vi "SDCP SMF Rx Logger - Test.vi"() -> ()   [LabVIEW 2020]
uses:
  Typedefs/SDCP SMF logger - SMF with timestamp.ctl
  SDCP SMF Rx Logger - FGV - Commands.vi
  Typedefs/SDCP - Serial Port Control - Commands.ctl
panel:
  out "Number of samples for instantaeneous samples":i32
  out "Instantaeneous logged data":T1[](array[typedef])
  out "Elapse time (ms)":u32
  out "Logging started":bool
  out "Number of samples":i32
  in  "Stop logging":bool
  in  "Log interval (ms)":u32
  in  "Number of iterations":i32
  out "Rx data":T1[](array[typedef])
  in  "Baud rate":u32=9600
  in  "COM Port":refnum<visa-resource-name>
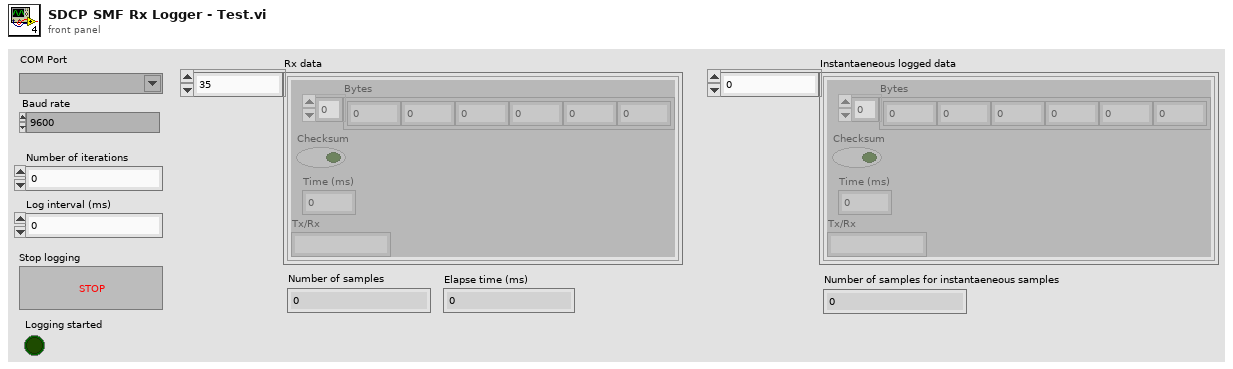
[diagram p1: front panel]
types:
  T1 = typedef "SDCP SMF logger - SMF with timestamp.ctl" = cluster{"Bytes":u8[], "Checksum":bool, "Time (ms)":u32, "Tx/Rx":string}
  T2 = typedef "SDCP - Serial Port Control - Commands.ctl" = enum16{"Open", "Read", "Write", "Get instance", "Close"}
  T3 = typedef "SDCP SMF Rx Logger - FGV - Commands.vi" = enum16{"Start logging", "Pause logging", "Get log data", "Reset log", "Stop logging"}
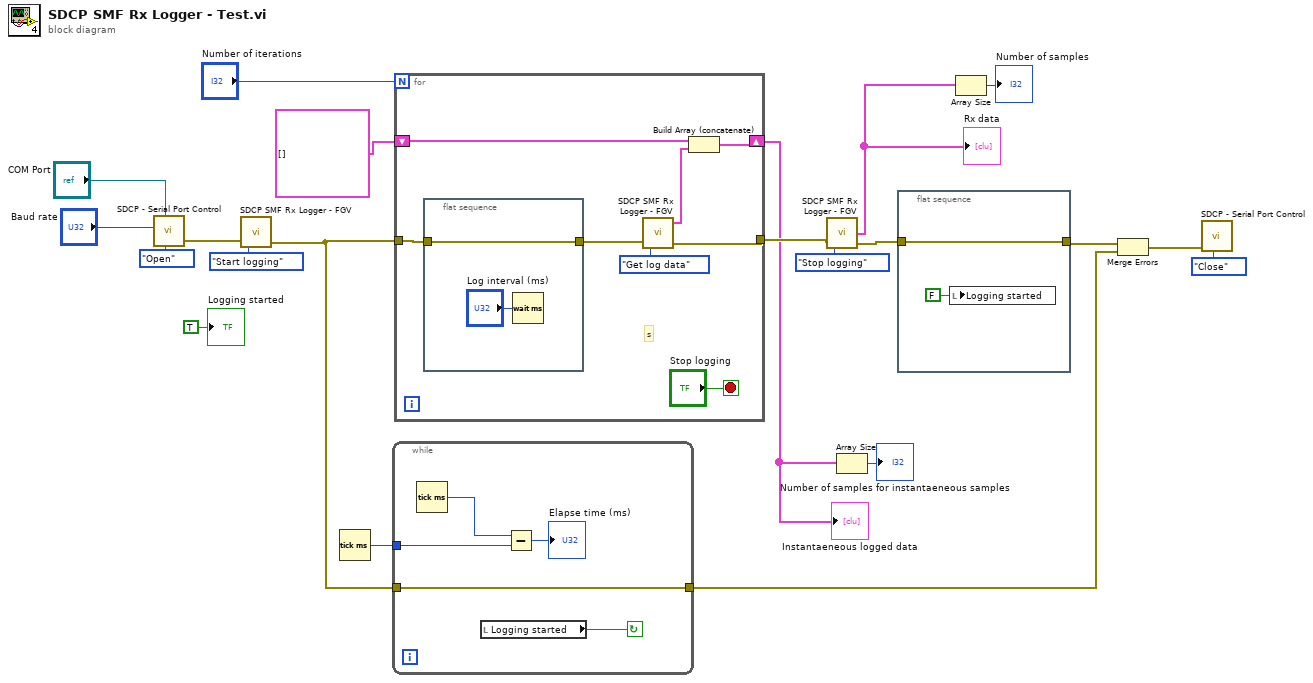
[diagram p0: block diagram]
diagram:
  n1 = call "SDCP - Serial Port Control.vi"("Command"=SDCP_-_Serial_Port_Control_-_Commands."Open", "VISA resource name"="COM Port", "Baud rate"="Baud rate") -> ("error out"=w19:errorcluster)  [unwired: 7 in, 1 out]
  n2 = call "SDCP SMF Rx Logger - FGV.vi"("Commands"=SDCP_SMF_Rx_Logger_-_FGV_-_Commands.vi."Start logging", "error in (no error)"=w19) -> ("error out"=w11:errorcluster)  [unwired: 2 out]
  n3 = Tick Count (ms)() -> (millisecond timer value=w5:u32)
  n4 = while {
    tunnel: w11 -> [w26]
    tunnel: [w26] -> w7
    tunnel: w5 -> [w24]
    stop <- w25 continue-if-true
    n5 = Tick Count (ms)() -> (millisecond timer value=w23:u32)
    n6 = local read "Logging started"() -> (w25:bool)
    n7 = Subtract(x=w23, y=w24) -> (x-y=→"Elapse time (ms)":u32)
  }
  n8 = for {
    N: "Number of iterations" -> [_]
    tunnel: w11 -> [w34]
    tunnel: [w31] -> w13
    shift-right: [w27] -> w1
    shift-left: T1[] [] ("Instantaeneous logged data") -> [w28]
    stop <- "Stop logging" stop-if-true
    # "s"
    n9 = flat-sequence {
      tunnel: w34 -> [w36]
      tunnel: [w36] -> w32
      frame #0 {
        n10 = Wait (ms)(milliseconds to wait="Log interval (ms)") -> ()  [unwired: 1 out]
      }
    }
    n11 = call "SDCP SMF Rx Logger - FGV.vi"("Commands"=SDCP_SMF_Rx_Logger_-_FGV_-_Commands.vi."Get log data", "error in (no error)"=w32) -> ("Instantaeneous logged data"=w29:T1[], "error out"=w31:errorcluster)  [unwired: 1 out]
    n12 = Build Array (concatenate)(w28, w29) -> (w27:T1[])
  }
  "Instantaeneous logged data" <- w1
  n13 = call "SDCP SMF Rx Logger - FGV.vi"("Commands"=SDCP_SMF_Rx_Logger_-_FGV_-_Commands.vi."Stop logging", "error in (no error)"=w13) -> ("Complete logged data"=w4:T1[], "error out"=w9:errorcluster)  [unwired: 1 out]
  "Rx data" <- w4
  n14 = Array Size(array=w1) -> (size(s)=→"Number of samples for instantaeneous samples":i32)
  n15 = flat-sequence {
    tunnel: w9 -> [w38]
    tunnel: [w38] -> w8
    frame #0 {
      n16 = local write "Logging started"(FALSE ("Logging started")) -> ()
    }
  }
  n17 = Array Size(array=w4) -> (size(s)=→"Number of samples":i32)
  n18 = Merge Errors(w8, w7) -> (w6:errorcluster)
  n19 = call "SDCP - Serial Port Control.vi"("Command"=SDCP_-_Serial_Port_Control_-_Commands."Close", "error in (no error)"=w6) -> ()  [unwired: 8 in, 2 out]
  "Logging started" <- TRUE ("Logging started")
